vi "fftGenX.vi"(10 "start":i32, 11 "Output Array":dbl[](array[numeric])) -> (3 "Array":i32[](array[numeric]))   [LabVIEW 2011]
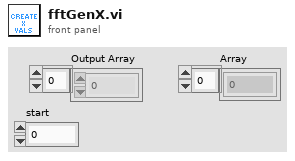
[diagram p1: front panel]
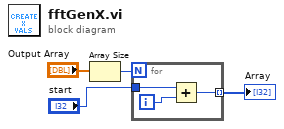
[diagram p0: block diagram]
diagram:
  n1 = Array Size(array="Output Array") -> (size(s)=w2:i32)
  n2 = for {
    N: w2 -> [_]
    tunnel: [w6] -> w3 mode=indexing
    tunnel: "start" -> [w5]
    i -> [w7]
    n3 = Add(x=w5, y=w7) -> (x+y=w6:i32)
  }
  "Array" <- w3
